vi "test data outputs.vi"() -> ()   [LabVIEW 2014]
panel:
  in  "testdata1":dbl[](array[numeric])
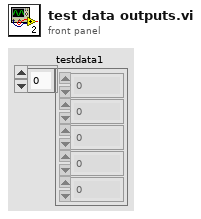
[diagram p1: front panel]
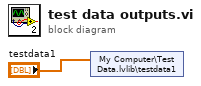
[diagram p0: block diagram]
diagram:
  n1 = shared-variable "My Computer\\Test Data.lvlib\\testdata1"("testdata1") -> ()  [unwired: 1 in, 1 out]
